vi "Start.vi"(8 "error in":errorcluster) -> (0 "error out":errorcluster)   [LabVIEW 2015, in "PLC.lvlib"]
uses:
  PLC.lvlib
  Solution/Production Line/support/Message Queue/Message Queue.lvlib
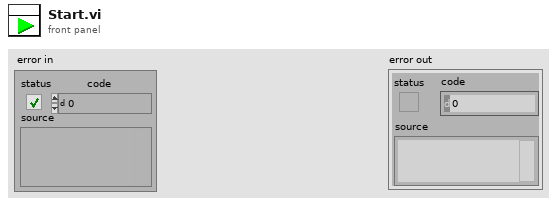
[diagram p1: front panel]
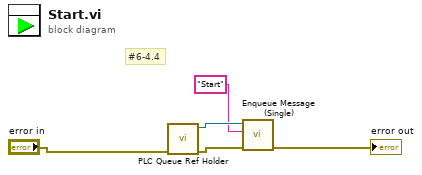
[diagram p0: block diagram]
diagram:
  # "#6-4.4"
  n1 = call "PLC Queue Ref Holder.vi"("error in"="error in") -> ("error out"=w3:errorcluster, "Input Message Queue"=w4:refnum<queue>)  [unwired: 9 in]
  n2 = call "Enqueue Message (Single).vi"("error in (no error)"=w3, "Message"="Start", "Message Queue"=w4) -> ("error out"=→"error out":errorcluster)  [unwired: 7 in, 1 out]
